vi "AT Get Enum Count A.vi"(8 "error in (no error)":errorcluster, 10 "Feature":string, 11 "Handle":i32) -> (0 "error out":errorcluster, 2 "Count":i32, 3 "Status":i32)   [LabVIEW 2019]
doc: "Get Enum Count\n\nReturn:\n I32 Status\n I32 Count\n\nParameters:\n I32 Handle\n String Feature\n\nThis function returns the number of indexes that the specified enumerated feature can be set to."
uses:
  atcoreA.dll
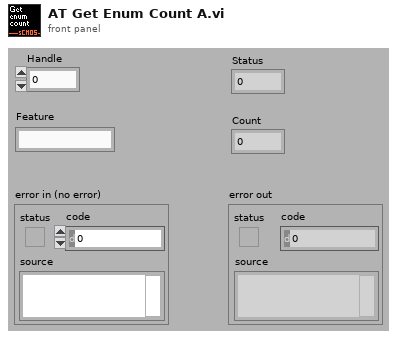
[diagram p1: front panel]
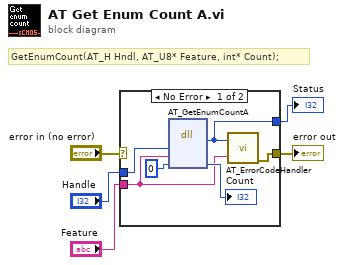
[diagram p0: block diagram]
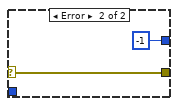
[diagram p2: hidden frame]
diagram:
  # "GetEnumCount(AT_H Hndl, AT_U8* Feature, int* Count);"
  n1 = case shown="No Error" "error in (no error)" {
    selector: "error in (no error)" -> [_ w13]
    tunnel: [w7 -1] -> w5
    tunnel: "Handle" -> [w11 _]
    tunnel: "Feature" -> [w6 _]
    tunnel: [w8 w13] -> w1
    frame No Error {
      n2 = dll-call lib="atcoreA.dll" fn="AT_GetEnumCountA"("Handle"=w11, "Feature"=w6, "Count"=0) -> ("Status"=w7:i32, "Count"=→"Count":i32)  [unwired: 5 in, 2 out]
      n3 = call <userlib>:"AT_ErrorCodeHandler.vi"("Error"=w7, "Feature Name"=w6) -> ("error out"=w8:errorcluster)  [unwired: 5 in]
    }
    frame Error {
    }
  }
  "Status" <- w5
  "error out" <- w1
